vi "ITX to LV 2.1 1D.vi"(8 "error in":errorcluster, 11 "file (use dialog)":path=path "P:/sample/GaAs/GaAs quantum dots/2008/PL Map/A1 735/060731ASBA_A1_6.0.itx") -> (0 "error out":errorcluster, 2 "1D arrays":dbl[][](array[numeric]), 3 "Data (Dictionary)":T1[](array[typedef]), 4 "Notes":string, 5 "base wavenames":string[](array[string]), 6 "Commands":string)   [LabVIEW 2016]
uses:
  Data.ITX.lvclass
  Data/Typedefs/Dictionary--cluster.ctl
  Data/Data.lvclass
panel:
  out "wavenames":string[](array[string])
  out "text to data":u32
  out "parse 2":u32
  out "parse 1 (ms)":u32
  out "open file (ms)":u32
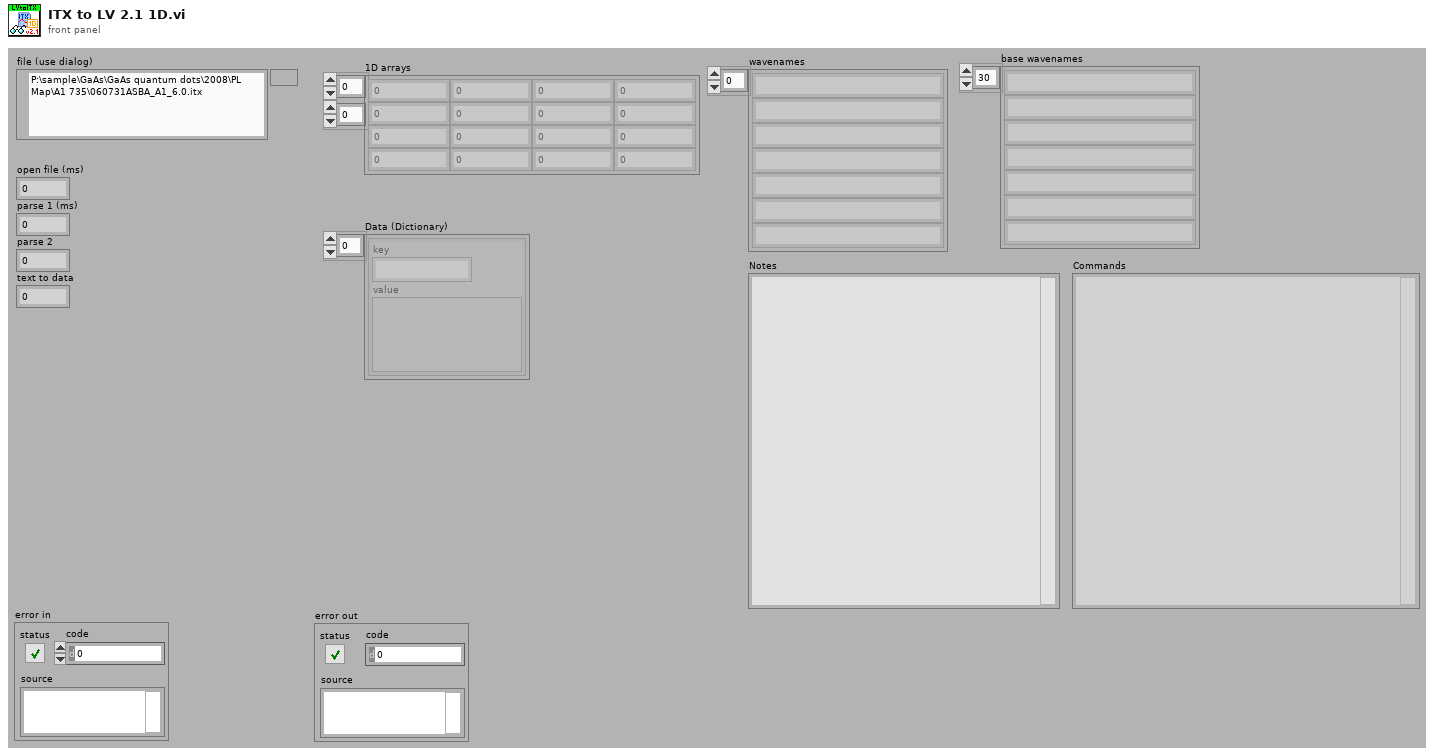
[diagram p1: front panel]
types:
  T1 = typedef "Data.lvclass/Dictionary--cluster.ctl" = cluster{"key":string, "value":variant}
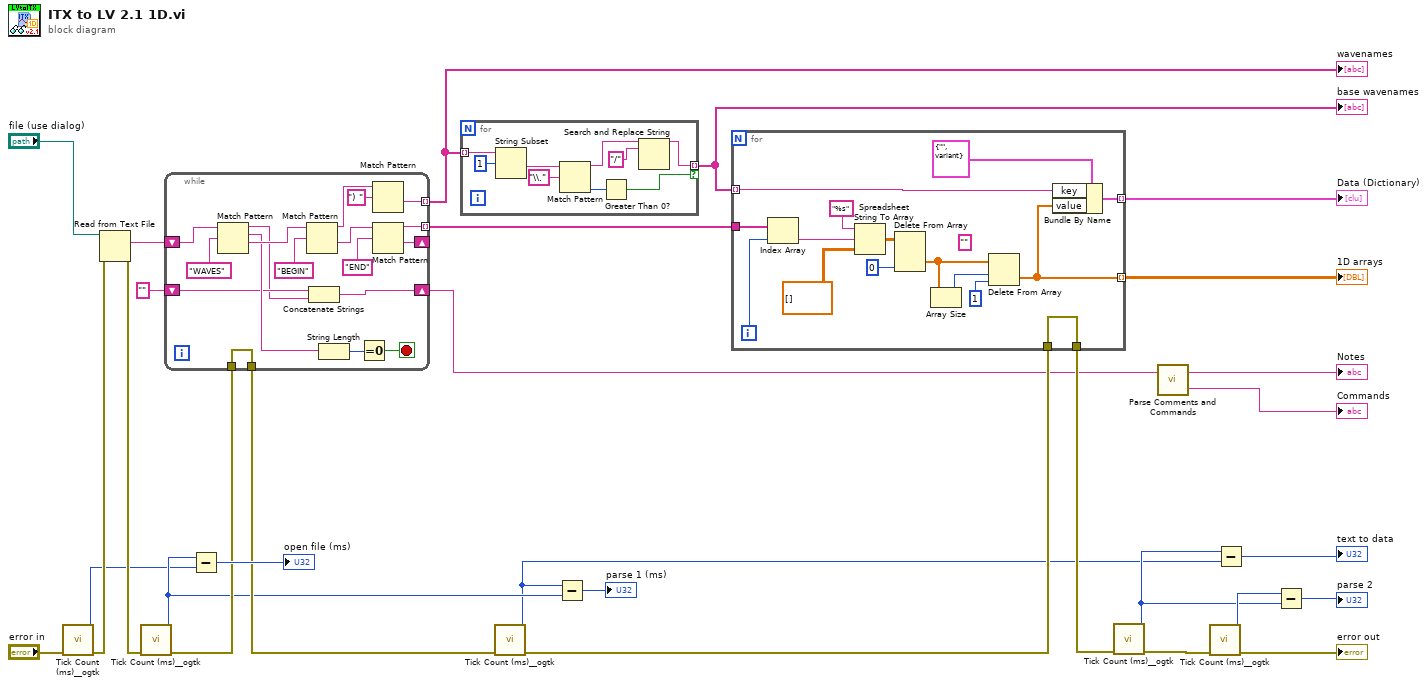
[diagram p0: block diagram]
diagram:
  n1 = call <userlib>:"Tick Count (ms)__ogtk.vi"("error in (no error)"="error in") -> ("error out"=w24:errorcluster, "millisecond timer value"=w3:u32)  [unwired: 9 in]
  n2 = Read from Text File(file (use dialog)="file (use dialog)", error in=w24) -> (text=w29:string, error out=w23:errorcluster)  [unwired: 1 in, 3 out]
  n3 = call <userlib>:"Tick Count (ms)__ogtk.vi"("error in (no error)"=w23) -> ("error out"=w17:errorcluster, "millisecond timer value"=w4:u32)  [unwired: 9 in]
  n4 = while {
    tunnel: [w31] -> w26 mode=indexing
    shift-right: [w45] -> _
    shift-left: w29 -> [w33]
    tunnel: [w41] -> w8 mode=indexing
    shift-right: [w36] -> w7
    shift-left: "" ("regular expression") -> [w35]
    tunnel: w17 -> [w30]
    tunnel: [w30] -> w12
    stop <- w42 stop-if-true
    n5 = Match Pattern(string=w33, regular expression="WAVES") -> (before substring=w34:string, match substring=w44:string, after substring=w47:string)  [unwired: 2 out]
    n6 = Match Pattern(string=w47, regular expression="BEGIN" ("regular expression 2")) -> (before substring=w32:string, after substring=w46:string)  [unwired: 3 out]
    n7 = Concatenate Strings(w35, w34) -> (w36:string)
    n8 = String Length(string=w44) -> (length=w43:i32)
    n9 = Equal To 0?(x=w43) -> (x = 0?=w42:bool)
    n10 = Match Pattern(string=w32, regular expression=") ") -> (after substring=w41:string)  [unwired: 4 out]
    n11 = Match Pattern(string=w46, regular expression="END" ("regular expression 3")) -> (before substring=w31:string, after substring=w45:string)  [unwired: 3 out]
  }
  "wavenames" <- w8
  n12 = Subtract(x=w4, y=w3) -> (x-y=→"open file (ms)":u32)
  n13 = for {
    tunnel: w8 -> [w55] mode=indexing
    tunnel: [w48] -> w9 mode=indexing if=w51
    n14 = String Subset(string=w55, offset (0)=1) -> (substring=w54:string)  [unwired: 1 in]
    n15 = Match Pattern(string=w54, regular expression="\\.") -> (before substring=w49:string, offset past match=w52:i32)  [unwired: 1 in, 2 out]
    n16 = Greater Than 0?(x=w52) -> (x > 0?=w51:bool)
    n17 = Search and Replace String(input string=w49, search string="/") -> (result string=w48:string)  [unwired: 6 in, 3 out]
  }
  "base wavenames" <- w9
  n18 = call <userlib>:"Tick Count (ms)__ogtk.vi"("error in (no error)"=w12) -> ("error out"=w16:errorcluster, "millisecond timer value"=w2:u32)  [unwired: 9 in]
  n19 = Subtract(x=w2, y=w4) -> (x-y=→"parse 1 (ms)":u32)
  n20 = for {
    tunnel: [w59] -> w28 mode=indexing
    tunnel: w26 -> [w66]
    tunnel: w16 -> [w61]
    tunnel: [w61] -> w13
    tunnel: w9 -> [w60] mode=indexing
    tunnel: [w58] -> w11 mode=indexing
    i -> [w63]
    (unwired) "" ("result string")
    n21 = Index Array(array=w66, index=w63) -> (element=w62:string)
    n22 = Spreadsheet String To Array(format string="%s", spreadsheet string=w62, array type (2D Dbl)=dbl[][] []) -> (array=w70:dbl[][])  [unwired: 1 out]
    n23 = Delete From Array(array=w70, index (col)=0 ("disabled index (col)")) -> (deleted portion=w69:dbl[])  [unwired: 2 in, 1 out]
    n24 = Array Size(array=w69) -> (size(s)=w68:i32)
    n25 = Delete From Array(array=w69, length=w68, index=1) -> (deleted portion=w59:dbl[])  [unwired: 1 out]
    n26 = Bundle By Name(cluster=T1 {"key"="", "value"=variant} ("key-value"), "key"=w60, "value"=w59) -> (w58:T1)
  }
  "1D arrays" <- w28
  "Data (Dictionary)" <- w11
  n27 = call <userlib>:"Tick Count (ms)__ogtk.vi"("error in (no error)"=w13) -> ("error out"=w1:errorcluster, "millisecond timer value"=w5:u32)  [unwired: 9 in]
  n28 = call "Parse Comments and Commands.vi"("ITX Notes and Commands"=w7) -> ("Commands"=→"Commands":string, "Notes"=→"Notes":string)  [unwired: 1 in]
  n29 = call <userlib>:"Tick Count (ms)__ogtk.vi"("error in (no error)"=w1) -> ("error out"=→"error out":errorcluster, "millisecond timer value"=w6:u32)  [unwired: 9 in]
  n30 = Subtract(x=w5, y=w2) -> (x-y=→"text to data":u32)
  n31 = Subtract(x=w6, y=w5) -> (x-y=→"parse 2":u32)
